vi "finalize_lib_tsmaster_win32.vi"(8 "错误输入（无错误）":errorcluster) -> (0 "错误输出":errorcluster)   [LabVIEW 2016]
uses:
  TSMaster.dll
panel:
  # "功能：\n结束同星CAN API的调用，并释放本调用方引起占用的驱动内存；\n不影响其他应用程序所占用的内存，即同时调用同一个硬件。"
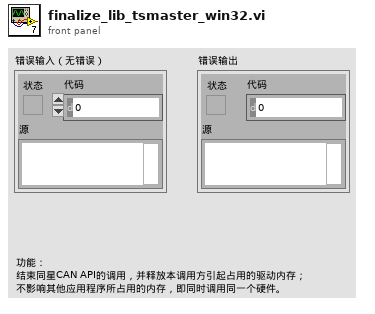
[diagram p1: front panel]
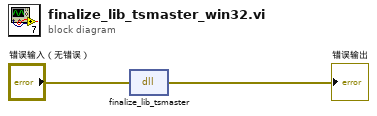
[diagram p0: block diagram]
diagram:
  n1 = dll-call lib="C:/Users/Eric/Desktop/LabVIEW/TSMasterAPI/Win32/CANopen_TS_2015/TSMaster.dll" fn="finalize_lib_tsmaster"(error in="错误输入（无错误）") -> (error out=→"错误输出":errorcluster)  [unwired: 3 in, 1 out]
